vi "nominal data values.vi"() -> ()   [LabVIEW 2018]
panel:
  out "Nominal Data Values":T1 {"%" format="%.2g"; "UW - VW VDC" format="%.2g"; "UV - VW VCD" format="%.2g"; "UV - UW VDC" format="%.2g"; "UW - VW L uH" format="%.2g"; "UV - VW L uH" format="%.2g"; "UV - UW L uH" format="%.2g"; "UW - VW mOhm" format="%.2g"; "UV - VW mOhm" format="%.2g"; "UV - UW mOhm" format="%.2g"; "back EMF VW VDC" format="%.2g"; "back EMF UW VDC" format="%.2g"; "back EMF UV VDC" format="%.2g"; "phase L VW uH" format="%.2g"; "phase L UW uH" format="%.2g"; "phase L UV uH" format="%.2g"; "phase R VW mOhm" format="%.2g"; "phase R UW mOhm" format="%.2g"; "phase R UV mOhm" format="%.2g"}
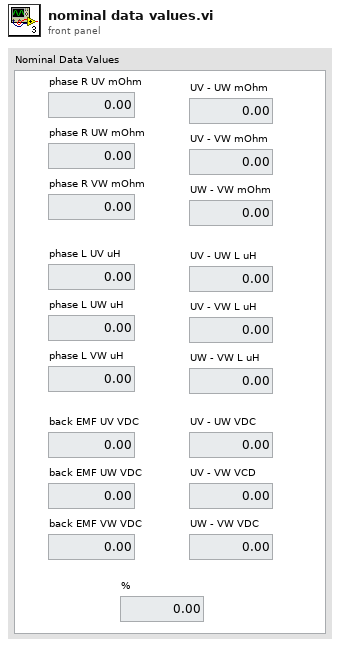
[diagram p1: front panel]
types:
  T1 = cluster{"phase R UV mOhm":dbl, "phase R UW mOhm":dbl, "phase R VW mOhm":dbl, "phase L UV uH":dbl, "phase L UW uH":dbl, "phase L VW uH":dbl, "back EMF UV VDC":dbl, "back EMF UW VDC":dbl, "back EMF VW VDC":dbl, "UV - UW mOhm":dbl, "UV - VW mOhm":dbl, "UW - VW mOhm":dbl, "UV - UW L uH":dbl, "UV - VW L uH":dbl, "UW - VW L uH":dbl, "UV - UW VDC":dbl, "UV - VW VCD":dbl, "UW - VW VDC":dbl, "%":dbl}
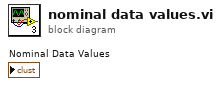
[diagram p0: block diagram]
diagram:
